vi "graphing_selection.vi"() -> ()   [LabVIEW 2017]
panel:
  in  "Tab Control":T1(tab)
  in  "TC Graph":T2
  out "TC Display":T3
  out "Waveform Chart":waveform(dbl)[](graph)=[{"t0"=timestamp(3580757854.087 s since 1904-01-01), "dt"=1.0, "Y"=[750.0616827041697]}, {"t0"=timestamp(3580757854.087 s since 1904-01-01), "dt"=1.0, "Y"=[750.0616827041697]}, {"t0"=timestamp(3580757854.087 s since 1904-01-01), "dt"=1.0, "Y"=[750.0616827041697]}]
  in  "Run 4":bool
  in  "Run 3":bool
  in  "Run 2":bool
  in  "Run":bool
  in  "Zone 2":T4 {"Zone Temp" items=["Average", "Maximum", "Minimum"]}
  out "Thermal Profile":dbl[](graph)
  in  "Zone 1":T4 {"Zone Temp" items=["Average", "Maximum", "Minimum"]}
  out "Custom Graphs 4":dbl[](graph)
  out "Custom Graphs 3":dbl[](graph)
  out "Custom Graphs 2":dbl[](graph)
  out "Custom Graphs":dbl[](graph)
  in  "stop":bool
  # "Set Point #"
  # "Temp goal"
  # "Soak Duration"
  # "Ramp"
  # "Set Point #"
  # "Temp goal"
  # "Soak Duration"
  # "Ramp"
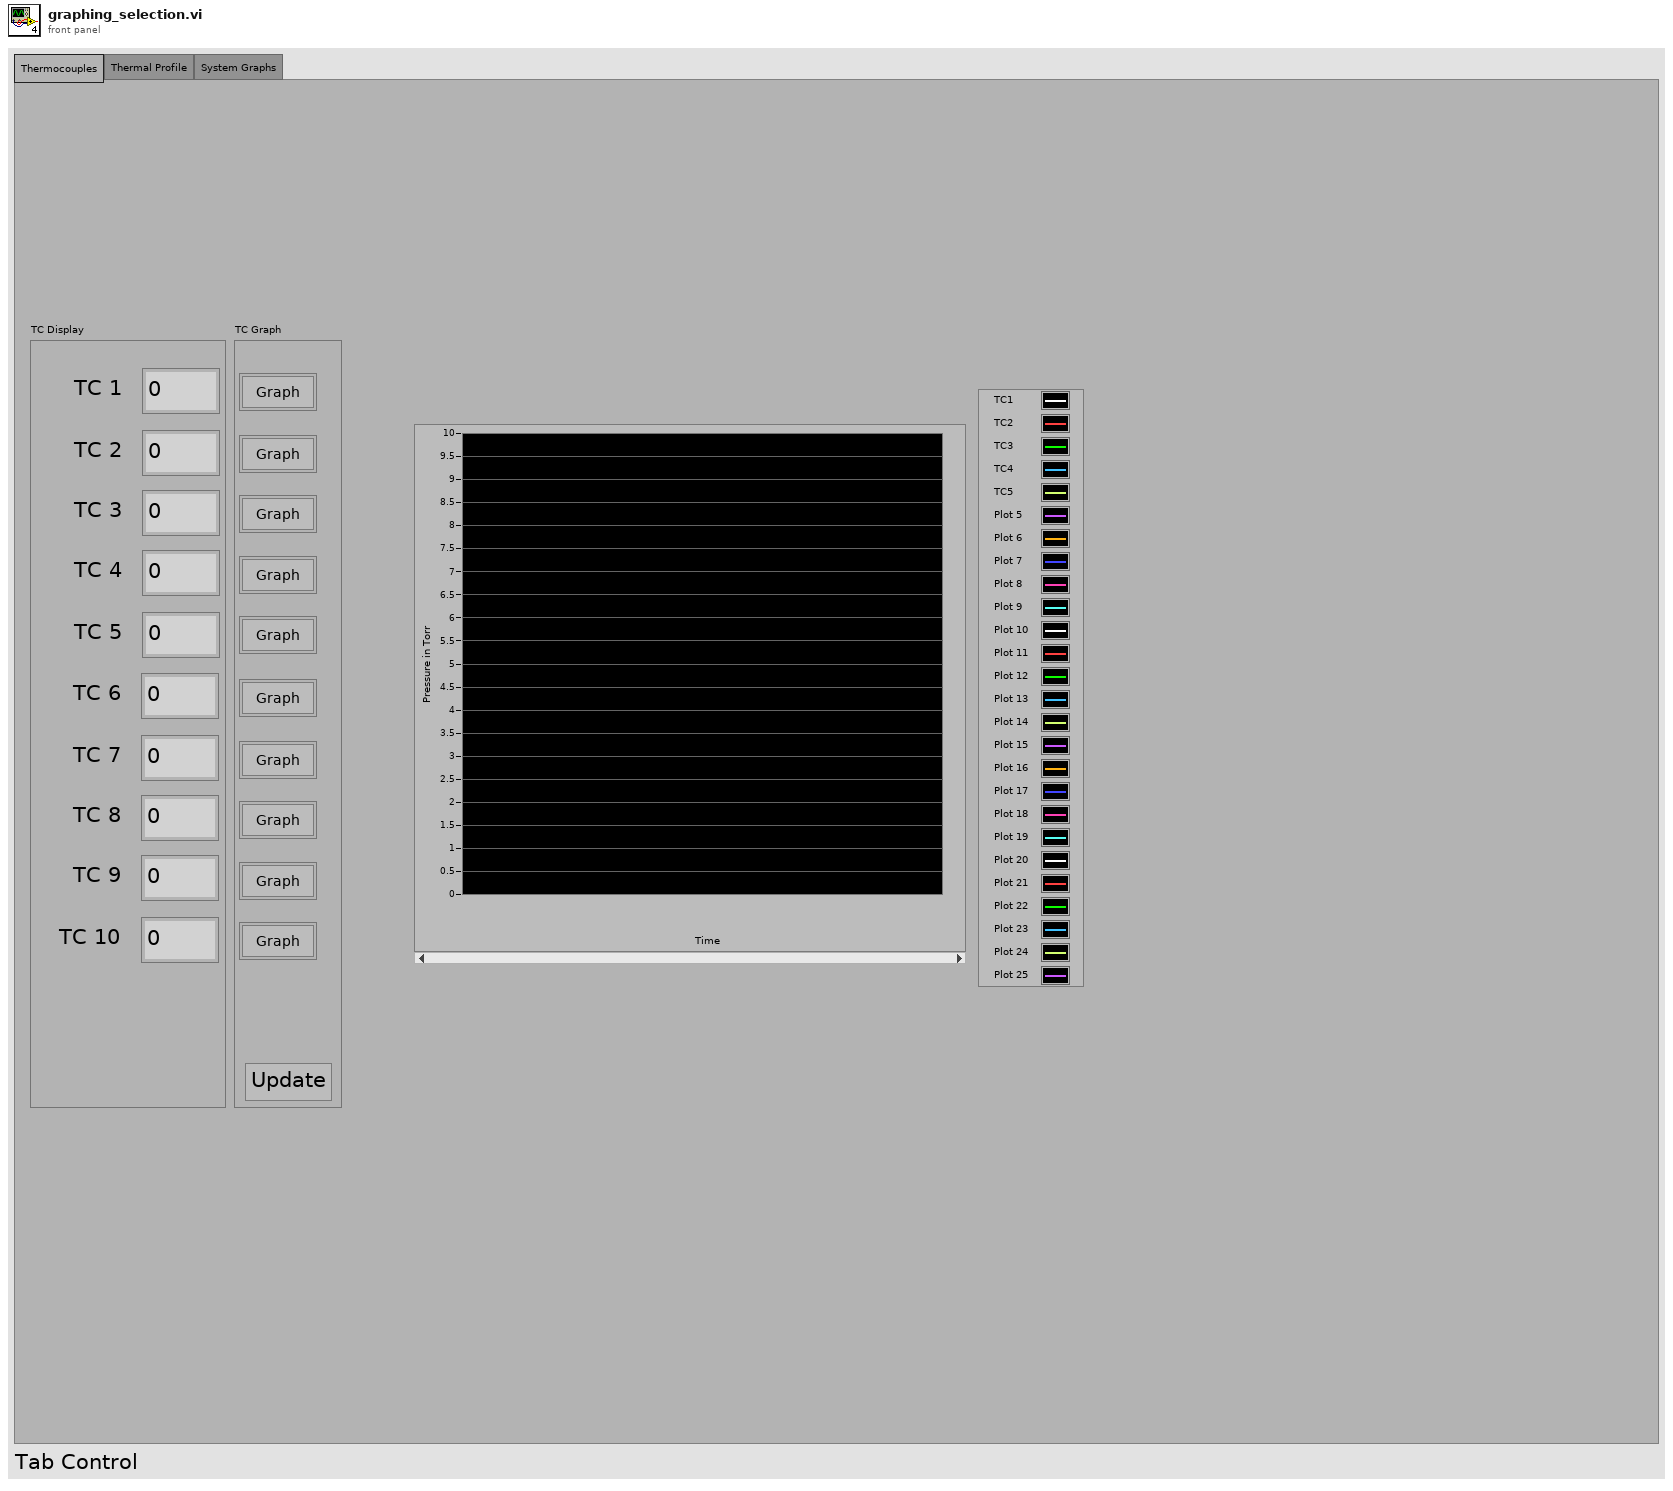
[diagram p1: front panel]
types:
  T1 = enum32{"Thermocouples", "Thermal Profile", "System Graphs"}
  T2 = cluster{"TC 1":bool, "TC 2":bool, "TC 3":bool, "TC 4":bool, "TC 5":bool, "Update":bool, "TC 6":bool, "TC 7":bool, "TC 8":bool, "TC 9":bool, "TC 10":bool}
  T3 = cluster{"TC 1":dbl, "TC 2":dbl, "TC 3":dbl, "TC 4":dbl, "TC 5":dbl, "TC 6":dbl, "TC 7":dbl, "TC 8":dbl, "TC 9":dbl, "TC 10":dbl}
  T4 = cluster{"Set Points":dbl[][], "Thermocouples in Zone":dbl[], "Zone Temp":u16}
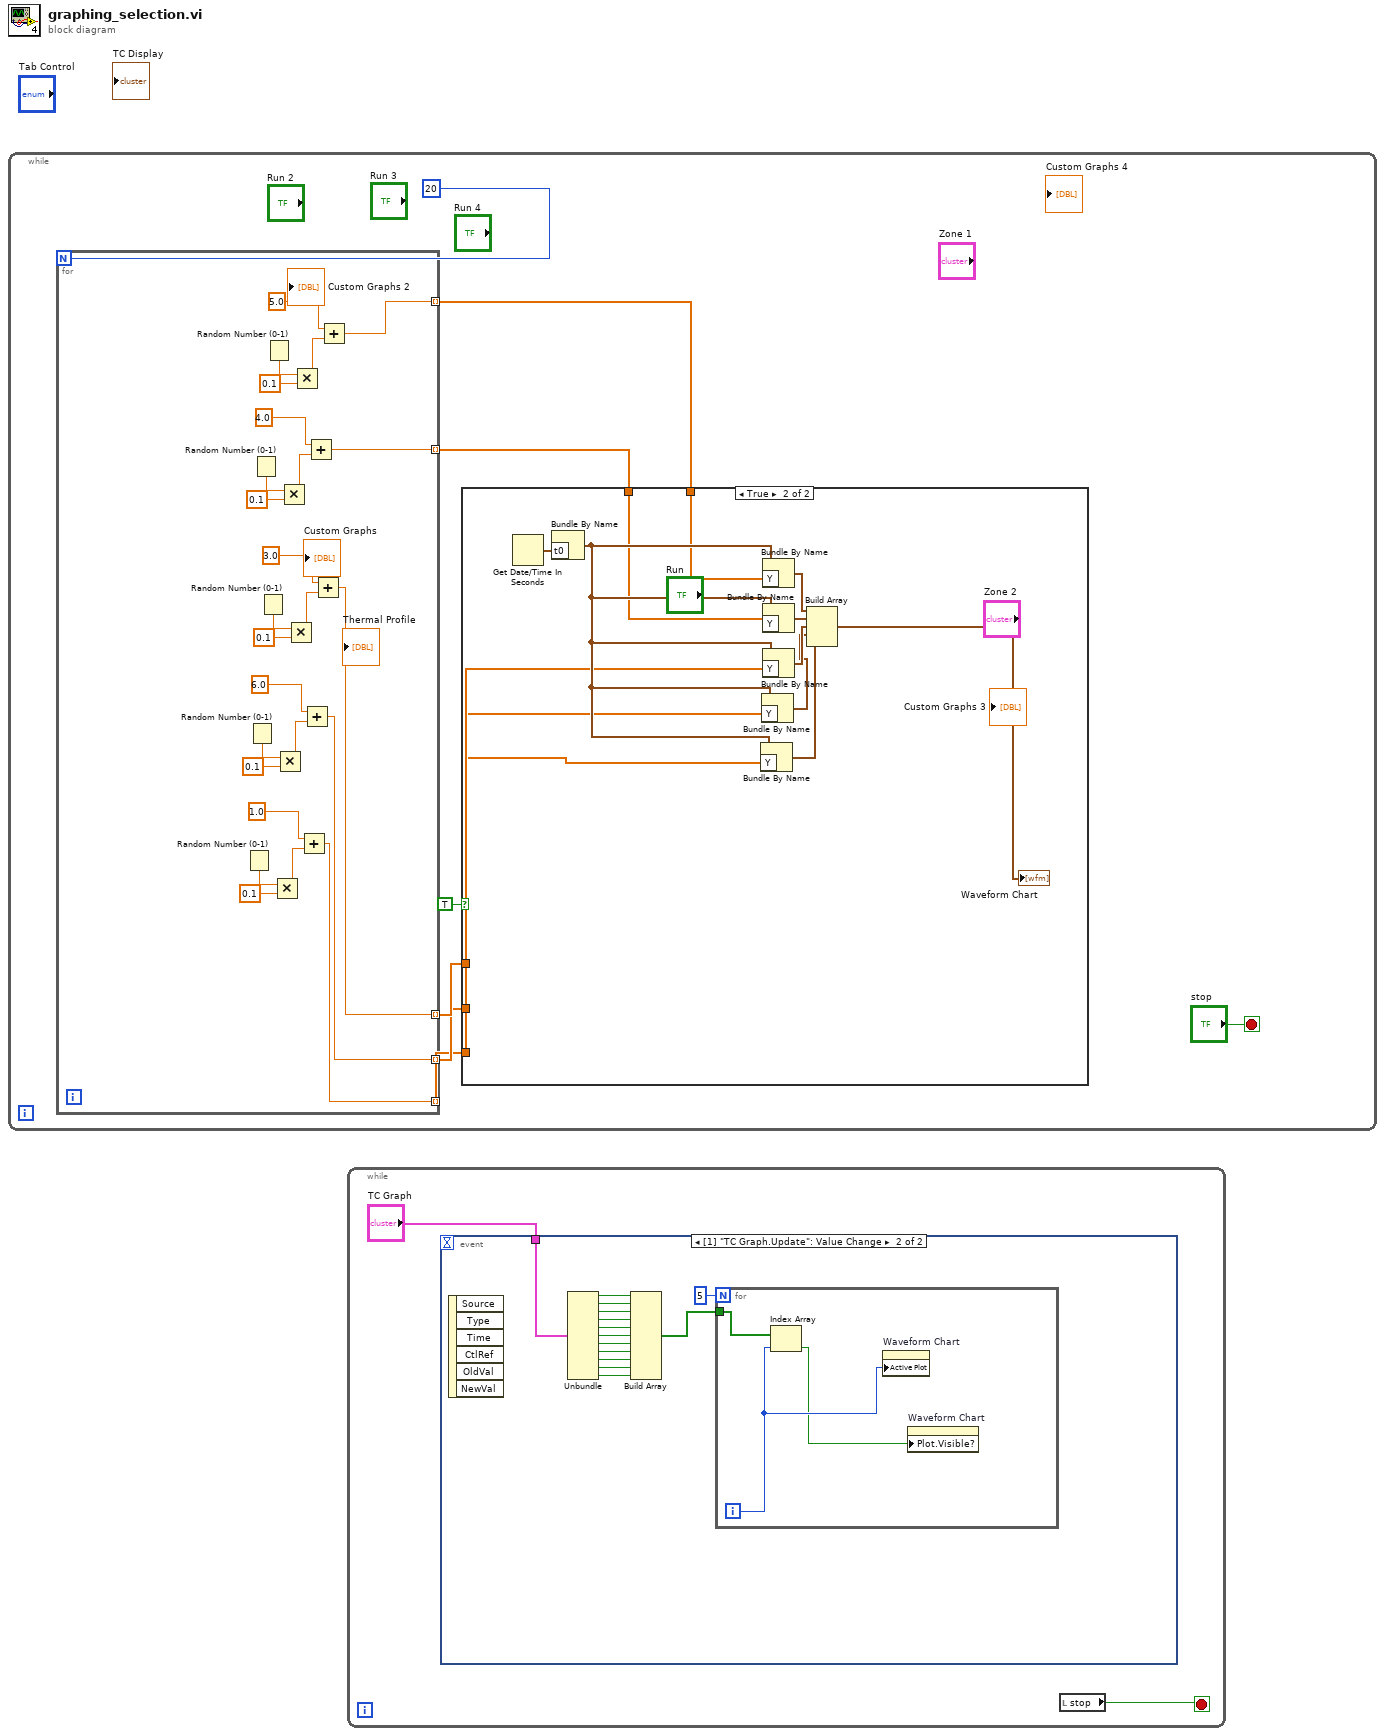
[diagram p0: block diagram]
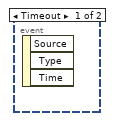
[diagram p2: hidden frame]
diagram:
  n1 = while {
    stop <- "stop" stop-if-true
    n2 = for {
      N: 20 -> [_]
      tunnel: [w42] -> w5 mode=indexing
      tunnel: [w25] -> w4 mode=indexing
      tunnel: [w24] -> w3 mode=indexing
      tunnel: [w23] -> w2 mode=indexing
      tunnel: [w22] -> w1 mode=indexing
      n3 = Random Number (0-1)() -> (number: 0 to 1=w33:dbl)
      n4 = Random Number (0-1)() -> (number: 0 to 1=w29:dbl)
      n5 = Random Number (0-1)() -> (number: 0 to 1=w41:dbl)
      n6 = Random Number (0-1)() -> (number: 0 to 1=w37:dbl)
      n7 = Random Number (0-1)() -> (number: 0 to 1=w46:dbl)
      n8 = Multiply(x=w33, y=0.1) -> (x*y=w31:dbl)
      n9 = Multiply(x=w29, y=0.1) -> (x*y=w27:dbl)
      n10 = Multiply(x=w41, y=0.1) -> (x*y=w39:dbl)
      n11 = Multiply(x=w37, y=0.1) -> (x*y=w35:dbl)
      n12 = Multiply(x=w46, y=0.1) -> (x*y=w44:dbl)
      n13 = Add(x=1.0 ("number (0 to 1)"), y=w31) -> (x+y=w22:dbl)
      n14 = Add(x=6.0 ("number (0 to 1)"), y=w27) -> (x+y=w23:dbl)
      n15 = Add(x=4.0 ("number (0 to 1)"), y=w39) -> (x+y=w25:dbl)
      n16 = Add(x=3.0 ("number (0 to 1)"), y=w35) -> (x+y=w24:dbl)
      n17 = Add(x=5.0 ("number (0 to 1)"), y=w44) -> (x+y=w42:dbl)
    }
    n18 = case shown="True" TRUE {
      tunnel: w5 -> [_ w13]
      tunnel: w4 -> [_ w12]
      tunnel: w3 -> [_ w11]
      tunnel: w2 -> [_ w10]
      tunnel: w1 -> [_ w9]
      frame False {
      }
      frame True {
        n19 = Get Date/Time In Seconds() -> (seconds since 1Jan1904=w21:timestamp)
        n20 = Bundle By Name("t0"=w21) -> (w14:waveform(dbl))  [unwired: 1 in]
        n21 = Bundle By Name(cluster=w14, "Y"=w9) -> (w15:waveform(dbl))
        n22 = Bundle By Name(cluster=w14, "Y"=w10) -> (w16:waveform(dbl))
        n23 = Bundle By Name(cluster=w14, "Y"=w13) -> (w20:waveform(dbl))
        n24 = Bundle By Name(cluster=w14, "Y"=w12) -> (w19:waveform(dbl))
        n25 = Bundle By Name(cluster=w14, "Y"=w11) -> (w18:waveform(dbl))
        n26 = Build Array(w20, w19, w18, w16, w15) -> (→"Waveform Chart":waveform(dbl)[])
      }
    }
  }
  n27 = while {
    stop <- w47 stop-if-true
    n28 = event shown="[1] \"TC Graph.Update\": Value Change" {
      selector: _ -> [_ _]
      dyn-events: _ -> [_ _]
      timeout: _ -> [_ _]
      tunnel: "TC Graph" -> [_ w62]
      event Timeout {
        n29 = event-data() -> ()  [unwired: 1 in, 3 out]
      }
      event "TC Graph.Update": Value Change {
        n30 = event-data() -> ()  [unwired: 1 in, 6 out]
        n31 = Unbundle(w62) -> ("TC 1"=w61:bool, "TC 2"=w60:bool, "TC 3"=w59:bool, "TC 4"=w58:bool, "TC 5"=w57:bool, "Update"=w54:bool, "TC 6"=w53:bool, "TC 7"=w52:bool, "TC 8"=w51:bool, "TC 9"=w50:bool, "TC 10"=w49:bool)
        n32 = Build Array(w61, w60, w59, w58, w57, w54, w53, w52, w51, w50, w49) -> (w56:bool[])
        n33 = for {
          N: 5 -> [_]
          tunnel: w56 -> [w65]
          i -> [w64]
          n34 = Index Array(array=w65, index=w64) -> (element=w63:bool)
          n35 = property on="Waveform Chart" class="WFChart (strict)"("Active Plot"=w64) -> ()  [unwired: 2 in, 2 out]
          n36 = property on="Waveform Chart" class="WFChart (strict)"("Plot.Visible?"=w63) -> ()  [unwired: 2 in, 2 out]
        }
      }
    }
    n37 = local read "stop"() -> (w47:bool)
  }
